vi "waveform_chart_prac.vi"() -> ()   [LabVIEW 2026]
panel:
  out "XY Graph":cluster{"X":dbl, "Y":dbl}[](graph)
  out "Waveform Graph":dbl[](graph)
  out "Waveform Chart":dbl(graph)
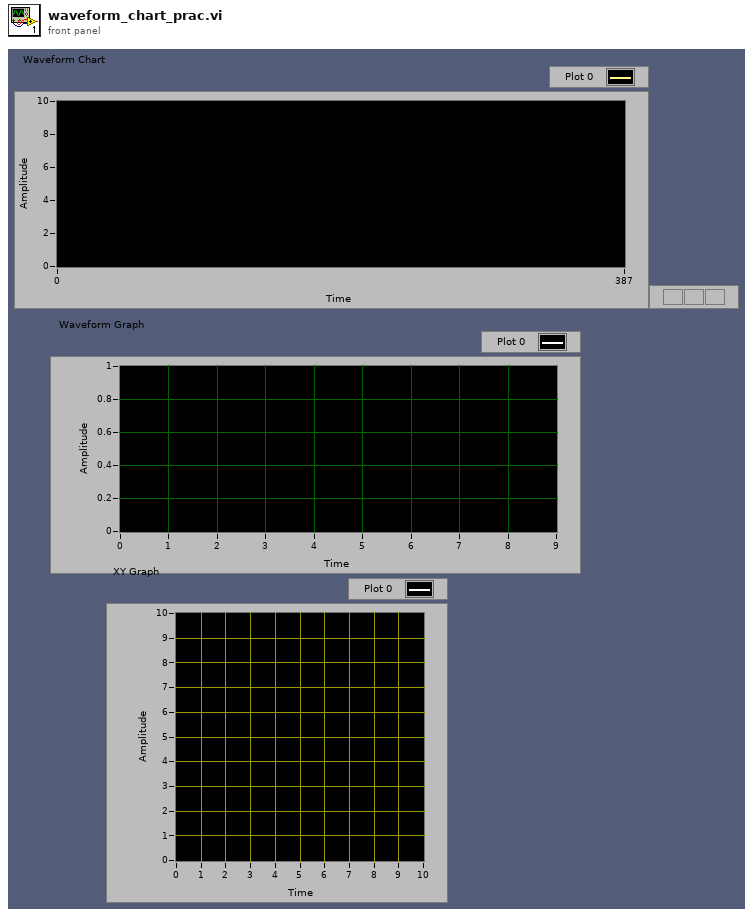
[diagram p1: front panel]
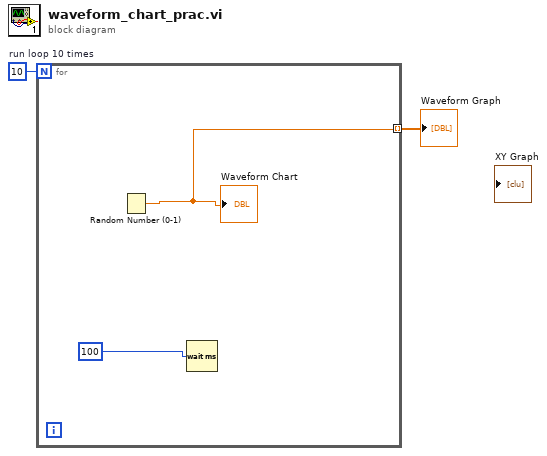
[diagram p0: block diagram]
diagram:
  w2 = 10  # run loop 10 times
  n1 = for {
    N: w2 -> [_]
    tunnel: [w3] -> w1 mode=indexing
    n2 = Random Number (0-1)() -> (number: 0 to 1=w3:dbl)
    "Waveform Chart" <- w3
    n3 = Wait (ms)(milliseconds to wait=100) -> ()  [unwired: 1 out]
  }
  "Waveform Graph" <- w1
